vi "GetFileCreationDate.vi"(9 "File Path":path) -> (0 "Error":bool, 3 "File Created Date (UTC)":timestamp)   [LabVIEW 2016]
uses:
  kernel32.dll
panel:
  in  "date time rec":T1
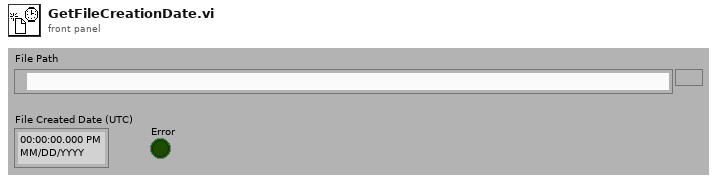
[diagram p1: front panel]
types:
  T1 = cluster{"fractional second":dbl, "second":i32, "minute":i32, "hour":i32, "day of month":i32, "month":i32, "year":i32, "day of week":i32, "day of year":i32, "DST":i32}
  T2 = cluster{"wYear":u16, "wMonth":u16, "wDayOfWeek":u16, "wDay":u16, "wHour":u16, "wMinute":u16, "wSeconds":u16, "wMilliseconds":u16}
  T3 = cluster{"dwFileAttributes":i32, "ftCreationTime":cluster{"dwLowDateTime":i32, "dwHighDateTime":i32}, "ftLastAccessTime":cluster{"dwLowDateTime":i32, "dwHighDateTime":i32}, "ftLastWrittenTime":cluster{"dwLowDateTime":i32, "dwHighDateTime":i32}, "nFileSizeHigh":i32, "nFileSizeLow":i32}
  T4 = cluster{"dwLowDateTime":i32, "dwHighDateTime":i32}
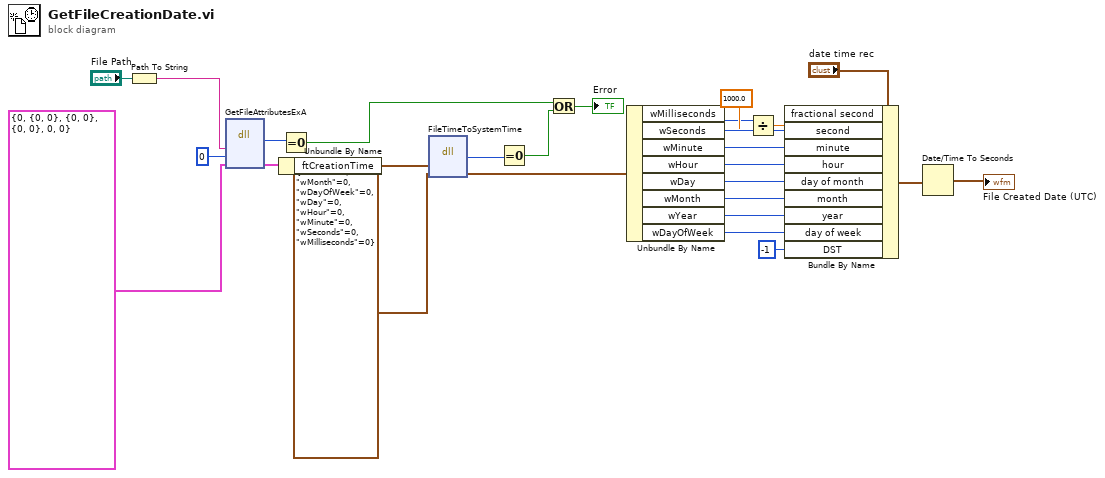
[diagram p0: block diagram]
diagram:
  n1 = Path To String(path="File Path") -> (string=w26:string)
  n2 = dll-call lib="kernel32.dll" fn="GetFileAttributesExA" label="GetFileAttributesEx"("lpFileName"=w26, "fInfoLevelID"=0, "output param"=T3 {"dwFileAttributes"=0, "ftCreationTime"={"dwLowDateTime"=0, "dwHighDateTime"=0}, "ftLastAccessTime"={"dwLowDateTime"=0, "dwHighDateTime"=0}, "ftLastWrittenTime"={"dwLowDateTime"=0, "dwHighDateTime"=0}, "nFileSizeHigh"=0, "nFileSizeLow"=0}) -> (w20:i32, "output param"=w23:T3)  [unwired: 5 in, 2 out]
  n3 = Unbundle By Name(w23) -> ("ftCreationTime"=w22:T4)
  n4 = Equal To 0?(x=w20) -> (x = 0?=w17:bool)
  n5 = dll-call lib="kernel32.dll" fn="FileTimeToSystemTime"("ftCreationTime"=w22, "output param"=T2 {"wYear"=0, "wMonth"=0, "wDayOfWeek"=0, "wDay"=0, "wHour"=0, "wMinute"=0, "wSeconds"=0, "wMilliseconds"=0}) -> (w19:i32, "output param"=w15:T2)  [unwired: 4 in, 2 out]
  n6 = Equal To 0?(x=w19) -> (x = 0?=w18:bool)
  n7 = Or(x=w17, y=w18) -> (x .or. y?=→"Error":bool)
  n8 = Unbundle By Name(w15) -> ("wMilliseconds"=w4:u16, "wSeconds"=w14:u16, "wMinute"=w13:u16, "wHour"=w12:u16, "wDay"=w11:u16, "wMonth"=w10:u16, "wYear"=w9:u16, "wDayOfWeek"=w8:u16)
  n9 = Divide(x=w4, y=1000.0) -> (x/y=w3:dbl)
  n10 = Bundle By Name(cluster="date time rec", "fractional second"=w3, "second"=w14, "minute"=w13, "hour"=w12, "day of month"=w11, "month"=w10, "year"=w9, "day of week"=w8, "DST"=-1) -> (w2:T1)
  n11 = Date/Time To Seconds(2:w2) -> (0:→"File Created Date (UTC)":timestamp)  [unwired: 1 in]
